vi "StageControl.vi"() -> ()   [LabVIEW 2014]
uses:
  <vilib>/Platform/TimedLoop/XDataNode/timing_clust.ctl
  <vilib>/Platform/TimedLoop/XDataNode/nitl_modes.ctl
  <vilib>/Platform/TimedLoop/XDataNode/wakeup.ctl
  <vilib>/FPGAPlugInAG/sbRIO-9632/niLvFpga_Open_sbRIO-9632.vi
  <vilib>/rvi/interface/common/dynamic/niFpgaDynamicAddResources.vi
  <vilib>/FPGAPlugInAG/Dynamic/niLvFpga_Reset_Dynamic.vi
  <vilib>/FPGAPlugInAG/Dynamic/niLvFpga_Download_Dynamic.vi
  <vilib>/FPGAPlugInAG/Dynamic/niLvFpga_Run_Dynamic.vi
  <vilib>/Utility/error.llb/Error Cluster From Error Code.vi
  <vilib>/rvi/errors/niLvFpgaAdjustHostInterfaceError.vi
  <vilib>/FPGAPlugInAG/Dynamic/niLvFpga_Close_Dynamic.vi
  <vilib>/rvi/interface/nirviOpenFPGA/nirviOpenFPGA.xnode
  FPGA Bitfiles/PPDControlLab3_FPGA_IP5.lvbitx
  SYSID_FPGA2.vi
  <vilib>/rvi/interface/nirviMethod/nirviMethod.xnode
  <vilib>/Platform/TimedLoop/XDataNode/XDataNode.xnode
  <vilib>/rvi/interface/nirviReadWriteControl/nirviReadWriteControl.xnode
  <vilib>/rvi/interface/nirviCloseFPGA/nirviCloseFPGA.xnode
  <vilib>/Platform/TimedLoop/XDataNode/XDNodeRunTimeDep.lvlib
  NiFpgaLv.dll
  <vilib>/rvi/interface/Simulation/niFpgaSimulationCallBeginRW.vi
panel:
  out "Right Limit":bool
  out "Left Limit":bool
  in  "Reset Position":bool
  in  "Enable Amplifier":bool
  in  "Start Control":bool
  out "Position (microns)":i32
  in  "Control (Volts)":fxp<+/-,20,5>
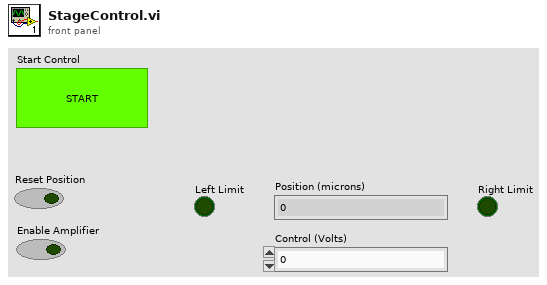
[diagram p1: front panel]
types:
  T1 = typedef "XDNodeRunTimeDep.lvlib/timing_clust.ctl" = cluster{"Expected End [f-1]":u64, "Actual End [f-1]":u64, "Finished Late? [f-1]":bool, "Expected End [i-1]":u64, "Actual End [i-1]":u64, "Finished Late? [i-1]":bool, "Expected Start [i]":u64, "Actual Start [i]":u64, "Expected Start [f]":u64, "Actual Start [f]":u64, "Source Name":string, "Structure Name":string, "Period":i64, "Deadline":i64, "Offset":i64, "Start":i64, "Priority":i32, "Timeout":i32, "Mode":T2, "Wakeup Reason":T3, "Error":errorcluster, "Source Type":string, "Secondary Source Type":string, "Global End Time":u64, "Global Start Time":u64, "Frame Duration":u64, "Iteration Duration":u64, "Assigned CPU":i32, "I/O Scan Engine Mode":u32}
  T2 = typedef "XDNodeRunTimeDep.lvlib/nitl_modes.ctl" = enum32{"No Change", "Process missed periods, maintain original phase", "Discard missed periods, maintain original phase", "Process missed periods, ignore original phase", "Discard missed periods, ignore original phase"}
  T3 = typedef "XDNodeRunTimeDep.lvlib/wakeup.ctl" = enum32{"Normal", "Aborted", "Asynchronous wakeup", "Timing source error", "Timed loop error", "Timeout"}
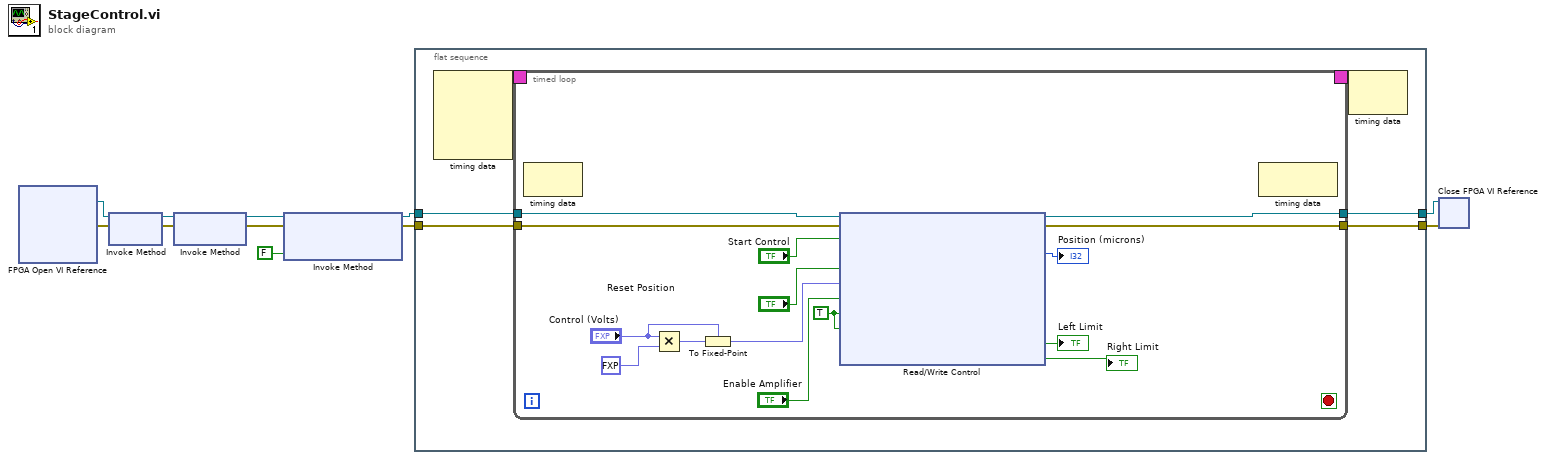
[diagram p0: block diagram]
diagram:
  n1 = xnode "FPGA Open VI Reference"() -> ("FPGA VI Reference Out"=w11:refnum<k20>, "error out"=w10:errorcluster)  [unwired: 2 in]
  n2 = xnode "Invoke Method"("FPGA VI Reference In"=w11, "error in"=w10) -> ("FPGA VI Reference Out"=w9:refnum<k20>, "error out"=w8:errorcluster)
  n3 = xnode "Invoke Method"("FPGA VI Reference In"=w9, "error in"=w8) -> ("FPGA VI Reference Out"=w7:refnum<k20>, "error out"=w6:errorcluster)
  n4 = xnode "Invoke Method"("FPGA VI Reference In"=w7, "error in"=w6, "Wait Until Done (F)"=FALSE) -> ("FPGA VI Reference Out"=w4:refnum<k20>, "error out"=w3:errorcluster)
  n5 = flat-sequence {
    tunnel: w4 -> [w15]
    tunnel: w3 -> [w14]
    tunnel: [w13] -> w2
    tunnel: [w12] -> w1
    frame #0 {
      n6 = node-c288() -> (w17:T1)  [unwired: 4 in]
      n7 = timed-loop {
        timing: w17 -> [_]
        timing-out: [_] -> w16
        tunnel: w15 -> [w32]
        tunnel: w14 -> [w31]
        tunnel: [w30] -> w13
        tunnel: [w29] -> w12
        stop <- _ stop-if-true
        w28 = TRUE ("Amp Reset")
        n8 = node-c288() -> ()  [unwired: 1 in, 1 out]
        n9 = Multiply(x="Control (Volts)", y=fxp<+/-,20,5> -1.0) -> (x*y=w20:fxp<+/-,40,10>)
        n10 = To Fixed-Point(fixed-point type="Control (Volts)", number=w20) -> (fixed-point=w18:fxp<+/-,20,5>)
        n11 = xnode "Read/Write Control"("FPGA VI Reference In"=w32, "error in"=w31, "Start 0"="Start Control", "quad reset (Port0/DIO0,Port0/DIO1)"="Reset Position", "State_Control"=w18, "Amp Enable"="Enable Amplifier", "Amp Reset"=w28, "Brake"=w28) -> ("FPGA VI Reference Out"=w30:refnum<k20>, "error out"=w29:errorcluster, "_quad pos (Port0/DIO0,Port0/DIO1)"=→"Position (microns)":i32, "Left Limit"=→"Left Limit":bool, "Right Limit"=→"Right Limit":bool)
        n12 = node-c288() -> ()  [unwired: 1 in, 1 out]
      }
      n13 = node-c288(w16) -> ()  [unwired: 1 out]
    }
  }
  n14 = xnode "Close FPGA VI Reference"("FPGA VI Reference In"=w2, "error in"=w1) -> ()  [unwired: 1 out]
